vi "Init.vi"(8 "error in (no error)":errorcluster, 10 "Node Reg":refnum<k20>, 11 "Case Structure in":refnum<class "Case Structure.lvclass">) -> (0 "error out":errorcluster, 3 "Case Structure out":refnum<class "Case Structure.lvclass">)   [LabVIEW 2025, in "Case Structure.lvclass"]
uses:
  Case Structure.lvclass
  C:/Users/mrjak/Documents/GitHub/LVGPT/LabVIEW/VIs/Classes/Node/Node.lvclass
  Controls/Tunnel.ctl
  Controls/Terminal.ctl
  Controls/wire.ctl
  Node.lvclass/Node.ctl
  MultiDiagramStructure.lvclass
  <vilib>/xml/NI_XML.lvlib
  Node.lvclass
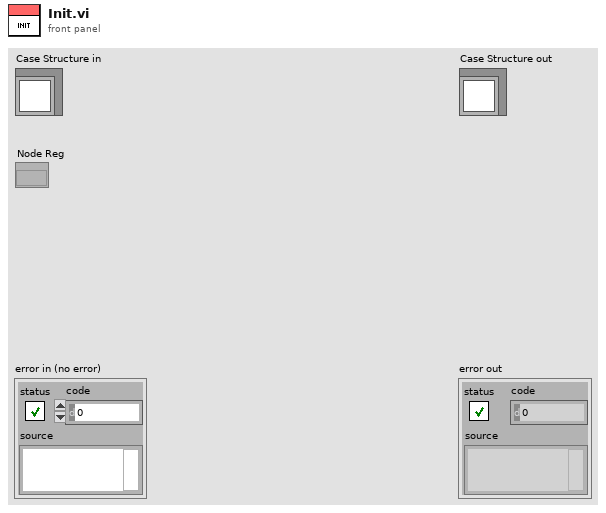
[diagram p1: front panel]
types:
  T1 = typedef "Terminal.ctl" = cluster{"id":string, "name":string, "terminal":refnum<vi>}
  T2 = typedef "Tunnel.ctl" = cluster{"OuterUUID":T1, "InnerUUIDs":T1[], "create_wire":T3}
  T3 = typedef "wire.ctl" = cluster{"id":string, "from":string, "to":string}
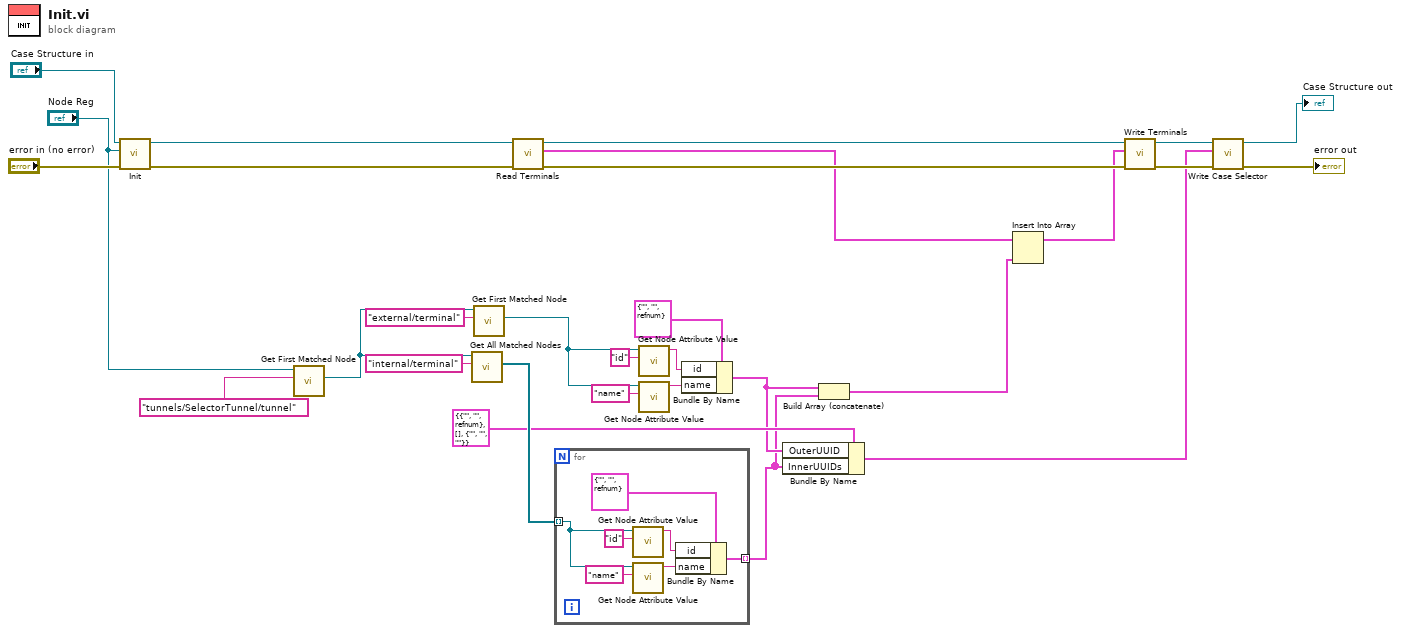
[diagram p0: block diagram]
diagram:
  n1 = call-parent "Init.vi"("error in (no error)"="error in (no error)", "Node Reg"="Node Reg", "Structure in"="Case Structure in") -> ("error out"=w12:errorcluster, "Structure out"=w11:refnum<class "Case Structure.lvclass">)  [unwired: 7 in]
  n2 = call <vilib>:"Get First Matched Node.vi"("XPath expression"="tunnels/SelectorTunnel/tunnel", "node in"="Node Reg") -> ("node result"=w13:refnum<k20>)  [unwired: 7 in, 2 out]
  n3 = call <vilib>:"Get All Matched Nodes.vi"("XPath expression"="internal/terminal", "node in"=w13) -> ("node result array"=w23:refnum<k20>[])  [unwired: 7 in, 2 out]
  n4 = call <vilib>:"Get First Matched Node.vi"("XPath expression"="external/terminal", "node in"=w13) -> ("node result"=w17:refnum<k20>)  [unwired: 7 in, 2 out]
  n5 = call "Read Terminals.vi"("error in (no error)"=w12, "Node in"=w11) -> ("error out"=w5:errorcluster, "Terminals"=w3:T1[], "Node out"=w4:refnum<class "Case Structure.lvclass">)  [unwired: 7 in]
  n6 = for {
    tunnel: w23 -> [w36] mode=indexing
    tunnel: [w30] -> w14 mode=indexing
    n7 = call "Get Node Attribute Value.vi"("Attribute Name"="id", "Refnum in"=w36) -> ("Value"=w31:string)  [unwired: 9 in]
    n8 = call "Get Node Attribute Value.vi"("Attribute Name"="name", "Refnum in"=w36) -> ("Value"=w32:string)  [unwired: 9 in]
    n9 = Bundle By Name(cluster=T1 {"id"="", "name"="", "terminal"=refnum} ("Terminal"), "id"=w31, "name"=w32) -> (w30:T1)
  }
  n10 = call "Get Node Attribute Value.vi"("Attribute Name"="id", "Refnum in"=w17) -> ("Value"=w18:string)  [unwired: 9 in]
  n11 = call "Get Node Attribute Value.vi"("Attribute Name"="name", "Refnum in"=w17) -> ("Value"=w19:string)  [unwired: 9 in]
  n12 = Bundle By Name(cluster=T1 {"id"="", "name"="", "terminal"=refnum} ("Terminal"), "id"=w18, "name"=w19) -> (w15:T1)
  n13 = Bundle By Name(cluster=T2 {"OuterUUID"={"id"="", "name"="", "terminal"=refnum}, "InnerUUIDs"=[], "create_wire"={"id"="", "from"="", "to"=""}} ("Tunnel"), "OuterUUID"=w15, "InnerUUIDs"=w14) -> (w7:T2)
  n14 = Build Array (concatenate)(w15, w14) -> (w1:T1[])
  n15 = Insert Into Array(array=w3, new element=w1) -> (w2:T1[])  [unwired: 1 in]
  n16 = call "Write Terminals.vi"("error in (no error)"=w5, "Terminals"=w2, "Node in"=w4) -> ("error out"=w10:errorcluster, "Node out"=w6:refnum<class "Case Structure.lvclass">)  [unwired: 7 in]
  n17 = call-dynamic "Write Case Selector.vi"("error in (no error)"=w10, "Tunnel"=w7, "Case Structure in"=w6) -> ("error out"=→"error out":errorcluster, "Case Structure out"=→"Case Structure out":refnum<class "Case Structure.lvclass">)  [unwired: 7 in]
